vi "Utility Format Flow Rate.vi"(8 "error in (no error)":errorcluster, 10 "Flow Rate":dbl, 11 "VISA resource name":refnum<visa-resource-name>) -> (0 "error out":errorcluster, 2 "Formatted Flow Rate":string, 3 "VISA resource name out":refnum<visa-resource-name>)   [LabVIEW 2020, in "ChromTech Series III Pump.lvlib"]
uses:
  ChromTech Series III Pump.lvlib
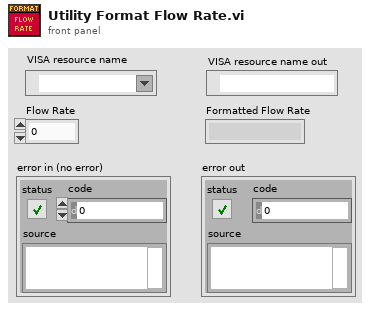
[diagram p1: front panel]
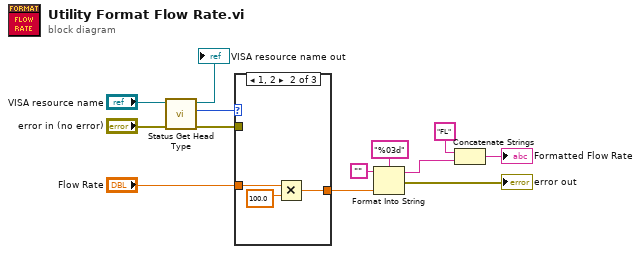
[diagram p0: block diagram]
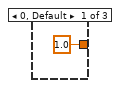
[diagram p2: hidden frame]
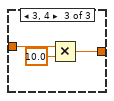
[diagram p3: hidden frame]
diagram:
  n1 = call "Status Get Head Type.vi"("error in"="error in (no error)", "VISA resource name"="VISA resource name") -> ("error out"=w9:errorcluster, "Head Type"=w10:i32, "VISA resource name out"=→"VISA resource name out":refnum<visa-resource-name>)  [unwired: 7 in]
  n2 = case shown="1, 2" w10 {
    tunnel: "Flow Rate" -> [_ w17 w19]
    tunnel: w9 -> [_ _ _]
    tunnel: [1.0 w15 w18] -> w5
    frame 0, Default {
    }
    frame 1, 2 {
      n3 = Multiply(x=w17, y=100.0) -> (x*y=w15:dbl)
    }
    frame 3, 4 {
      n4 = Multiply(x=w19, y=10.0) -> (x*y=w18:dbl)
    }
  }
  n5 = Format Into String(format string="%03d", initial string="", w5) -> (resulting string=w4:string, error out=→"error out":errorcluster)  [unwired: 1 in]
  n6 = Concatenate Strings("FL" ("string"), w4) -> (→"Formatted Flow Rate":string)
